vi "LVClass_Image ctor load.vi"(0 "Image (const)":refnum<class "Image.lvclass">, 7 "himg path":path, 11 "error in (no error)":errorcluster) -> (4 "Image (new)":refnum<class "Image.lvclass">, 15 "error out":errorcluster)   [LabVIEW 2020, in "Image.lvclass"]
doc: "Image constructor from file.\n\n--------------------------------------------------------------------------------\n\n<B>ImageIn</B> : Constant Pointer to Image object.\n<B>ImageOut</B> : Pointer to Image object.\n<B>image_file_path</B> : Absolute path to image file.\n<B>ErrorIn</B> : Error\n<B>ErrorOut</B> : Error\n\n--------------------------------------------------------------------------------"
uses:
  Image.lvclass
  Controls/Handle creation.ctl
  Image.lvclass/Image.ctl
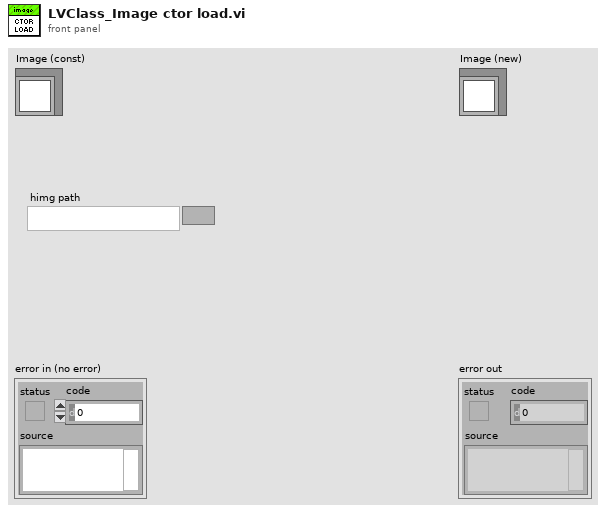
[diagram p1: front panel]
types:
  T1 = typedef "Handle creation.ctl" = enum16{"By ctor", "By write function"}
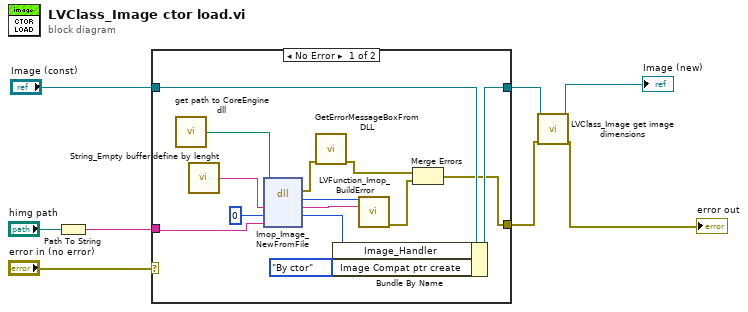
[diagram p0: block diagram]
diagram:
  n1 = Path To String(path="himg path") -> (string=w5:string)
  n2 = case shown="No Error" "error in (no error)" {
    selector: "error in (no error)" -> [_ w24]
    tunnel: [w9 w24] -> w4
    tunnel: [w17 w23] -> w2
    tunnel: "Image (const)" -> [w18 w23]
    tunnel: w5 -> [w13 _]
    frame No Error {
      n3 = call "get path to CoreEngine dll.vi"() -> ("path to wavekit library"=w15:path)  [unwired: 14 in, 1 out]
      n4 = call "String_Empty buffer define by lenght.vi"() -> ("Empty buffer"=w20:string)  [unwired: 1 in]
      n5 = dll-call lib="D:/soft/HASO_v3/SVN_trunk/ImOpCoreEngine4_LV2011/DLLs/c_interface_vc100.dll" fn="Imop_Image_NewFromFile"(path in=w15, "message"=w20, "Image compat"=0, "path"=w13) -> (error out=w14:errorcluster, "return type"=w21:i32, "message"=w22:string, "Image compat"=w19:i64)  [unwired: 3 in, 1 out]
      n6 = call "GetErrorMessageBoxFromDLL.vi"("error IN"=w14) -> ("error OUT"=w11:errorcluster)  [unwired: 10 in]
      n7 = Bundle By Name(cluster=w18, "Image_Handler"=w19, "Image Compat ptr create"=Handle_creation."By ctor") -> (w17:refnum<class "Image.lvclass">)
      n8 = call "LVFunction_Imop_BuildError.vi"("code"=w21, "String to Prepend to source (\"\")"=w22) -> ("error out"=w10:errorcluster)  [unwired: 13 in]
      n9 = Merge Errors(w11, w10) -> (w9:errorcluster)
    }
    frame Error {
    }
  }
  n10 = call "LVClass_Image get image dimensions.vi"("Image in"=w2, "error in (no error)"=w4) -> ("Image out"=→"Image (new)":refnum<class "Image.lvclass">, "error out"=→"error out":errorcluster)  [unwired: 10 in, 2 out]
